vi "dfd_Rotate FIR Direct.vi"(5 "#taps per phase":i32, 9 "state idx":T1={"start"=0, "stepsize"=1}, 10 "state in":i64[](array[numeric]), 11 "x":i64) -> (2 "state out":i64[](array[numeric]))   [LabVIEW 2017, in "NI_DigFilter_FXP.lvlib"]
uses:
  <vilib>/addons/Digital Filter Design/NI_DigFilter_FXP.lvlib
  <vilib>/addons/Digital Filter Design/_Objects.llb/dfd_Index Config.ctl
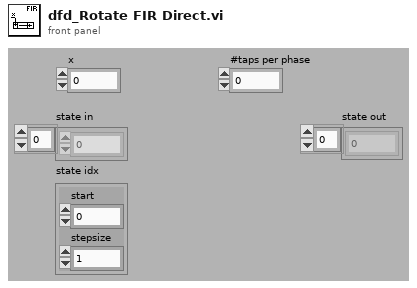
[diagram p1: front panel]
types:
  T1 = typedef "dfd_Index Config.ctl" = cluster{"start":i32, "stepsize":i32}
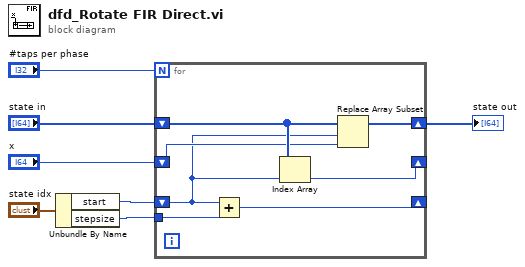
[diagram p0: block diagram]
diagram:
  n1 = Unbundle By Name("state idx") -> ("start"=w5:i32, "stepsize"=w4:i32)
  n2 = for {
    N: "#taps per phase" -> [_]
    shift-right: [w11] -> w2
    shift-left: "state in" -> [w13]
    shift-right: [w12] -> _
    shift-left: w5 -> [w9]
    tunnel: w4 -> [w14]
    shift-right: [w8] -> _
    shift-left: "x" -> [w10]
    n3 = Add(x=w9, y=w14) -> (x+y=w12:i32)
    n4 = Index Array(array=w13, index=w9) -> (element=w8:i64)
    n5 = Replace Array Subset(array=w13, new element=w10, index=w9) -> (w11:i64[])
  }
  "state out" <- w2
